vi "Test Asic Digital Offset.vi"(8 "Error IN":errorcluster, 11 "Config Test IN":T4={"Config HW"={"VISA Rigol DP832"="Rigol_DP832", "Config Rigol DP832"=[{"Channel"=0, "V Limit"=5.5, "I Limit"=0.5, "V Out"=5.0}, {"Channel"=1, "V Limit"=5.5, "I Limit"=0.8, "V Out"=5.0}, {"Channel"=2, "V Limit"=5.5, "I Limit"=0.2, "V Out"=0.0}], "CTA Test#"="CTA013 A", "FT_Handle"=0, "Espera acceso FT"=10, "VISA Tek MDO3104"="Rigol_DP832", "VISA Key 81160A"="Rigol_DP832"}, "Config Test"=[{"Vasic"=2.8, "Global Reset"=FALSE, "Test Register?"=FALSE, "Test ADC?"=FALSE, "Test ADC"={"Repeats ADC"=100, "Max Desviation"=0.1}, "Limits ADC"={"Low"=[1.9, 1.3, 0.65, 0.0, 1.6, 1.4, 1.4, 0.9, 2.1, 0.85, 1.9], "High"=[2.1, 1.5, 0.85, 0.1, 1.4, 1.2, 1.2, 0.7, 1.9, 0.65, 1.7]}, "Test Max PN Min NP?"=FALSE, "Limits Max PN Min NP"={"Max P Upper"=2.177000045776367, "Min P Upper"=1.474, "Max N Upper"=1.475, "Min N Upper"=0.818, "Max P Lower"=1.888, "Min P Lower "=1.321, "Max N Lower"=1.322, "Min N Lower"=0.73}, "Test Rate Scan?"=FALSE, "Vin Rate Scan"=[], "Limits Rate Scan"={"High"=[0.15, 0.242, 0.331, 0.425, 0.512, 0.6, 0.688, 0.774, 0.847, 0.91], "Low"=[0.021, 0.11, 0.189, 0.27, 0.347, 0.421, 0.487, 0.551, 0.601, 0.635]}, "Test Rate Scan Adders?"=FALSE, "Vin Rate Adders"=[], "Limits Rate Scan adders"={"High"=[], "Low"=[]}, "Test offset analog?"=FALSE, "Lim Offset Analog"={"Max Analog"=0.05, "Min Analog"=-0.05}, "Test offset digital?"=FALSE, "Lim offset Dig"={"Max Dig"=0.05}, "Vasic real f.a."=2.8, "IBIAS"=FALSE, "VALUE IBIAS"=63}, {"Vasic"=2.8, "Global Reset"=FALSE, "Test Register?"=FALSE, "Test ADC?"=FALSE, "Test ADC"={"Repeats ADC"=100, "Max Desviation"=0.1}, "Limits ADC"={"Low"=[1.9, 1.3, 0.65, 0.0, 1.6, 1.4, 1.4, 0.9, 2.1, 0.85, 1.9], "High"=[2.1, 1.5, 0.85, 0.1, 1.4, 1.2, 1.2, 0.7, 1.9, 0.65, 1.7]}, "Test Max PN Min NP?"=FALSE, "Limits Max PN Min NP"={"Max P Upper"=2.177000045776367, "Min P Upper"=1.474, "Max N Upper"=1.475, "Min N Upper"=0.818, "Max P Lower"=1.888, "Min P Lower "=1.321, "Max N Lower"=1.322, "Min N Lower"=0.73}, "Test Rate Scan?"=FALSE, "Vin Rate Scan"=[], "Limits Rate Scan"={"High"=[0.15, 0.242, 0.331, 0.425, 0.512, 0.6, 0.688, 0.774, 0.847, 0.91], "Low"=[0.021, 0.11, 0.189, 0.27, 0.347, 0.421, 0.487, 0.551, 0.601, 0.635]}, "Test Rate Scan Adders?"=FALSE, "Vin Rate Adders"=[], "Limits Rate Scan adders"={"High"=[], "Low"=[]}, "Test offset analog?"=FALSE, "Lim Offset Analog"={"Max Analog"=0.05, "Min Analog"=-0.05}, "Test offset digital?"=FALSE, "Lim offset Dig"={"Max Dig"=0.05}, "Vasic real f.a."=2.8, "IBIAS"=FALSE, "VALUE IBIAS"=63}, {"Vasic"=2.8, "Global Reset"=FALSE, "Test Register?"=FALSE, "Test ADC?"=FALSE, "Test ADC"={"Repeats ADC"=100, "Max Desviation"=0.1}, "Limits ADC"={"Low"=[1.9, 1.3, 0.65, 0.0, 1.6, 1.4, 1.4, 0.9, 2.1, 0.85, 1.9], "High"=[2.1, 1.5, 0.85, 0.1, 1.4, 1.2, 1.2, 0.7, 1.9, 0.65, 1.7]}, "Test Max PN Min NP?"=FALSE, "Limits Max PN Min NP"={"Max P Upper"=2.177000045776367, "Min P Upper"=1.474, "Max N Upper"=1.475, "Min N Upper"=0.818, "Max P Lower"=1.888, "Min P Lower "=1.321, "Max N Lower"=1.322, "Min N Lower"=0.73}, "Test Rate Scan?"=FALSE, "Vin Rate Scan"=[], "Limits Rate Scan"={"High"=[0.15, 0.242, 0.331, 0.425, 0.512, 0.6, 0.688, 0.774, 0.847, 0.91], "Low"=[0.021, 0.11, 0.189, 0.27, 0.347, 0.421, 0.487, 0.551, 0.601, 0.635]}, "Test Rate Scan Adders?"=FALSE, "Vin Rate Adders"=[], "Limits Rate Scan adders"={"High"=[], "Low"=[]}, "Test offset analog?"=FALSE, "Lim Offset Analog"={"Max Analog"=0.05, "Min Analog"=-0.05}, "Test offset digital?"=FALSE, "Lim offset Dig"={"Max Dig"=0.05}, "Vasic real f.a."=2.8, "IBIAS"=FALSE, "VALUE IBIAS"=63}, {"Vasic"=2.8, "Global Reset"=FALSE, "Test Register?"=FALSE, "Test ADC?"=FALSE, "Test ADC"={"Repeats ADC"=100, "Max Desviation"=0.1}, "Limits ADC"={"Low"=[1.9, 1.3, 0.65, 0.0, 1.6, 1.4, 1.4, 0.9, 2.1, 0.85, 1.9], "High"=[2.1, 1.5, 0.85, 0.1, 1.4, 1.2, 1.2, 0.7, 1.9, 0.65, 1.7]}, "Test Max PN Min NP?"=FALSE, "Limits Max PN Min NP"={"Max P Upper"=2.177000045776367, "Min P Upper"=1.474, "Max N Upper"=1.475, "Min N Upper"=0.818, "Max P Lower"=1.888, "Min P Lower "=1.321, "Max N Lower"=1.322, "Min N Lower"=0.73}, "Test Rate Scan?"=FALSE, "Vin Rate Scan"=[], "Limits Rate Scan"={"High"=[0.15, 0.242, 0.331, 0.425, 0.512, 0.6, 0.688, 0.774, 0.847, 0.91], "Low"=[0.021, 0.11, 0.189, 0.27, 0.347, 0.421, 0.487, 0.551, 0.601, 0.635]}, "Test Rate Scan Adders?"=FALSE, "Vin Rate Adders"=[], "Limits Rate Scan adders"={"High"=[], "Low"=[]}, "Test offset analog?"=FALSE, "Lim Offset Analog"={"Max Analog"=0.05, "Min Analog"=-0.05}, "Test offset digital?"=FALSE, "Lim offset Dig"={"Max Dig"=0.05}, "Vasic real f.a."=2.8, "IBIAS"=FALSE, "VALUE IBIAS"=63}], "Result"=[], "Execucion Test"={"Vasic Actual"=0}, "Config VGA"={"Theoretical Voltage"=[], "Real Voltage"=[102.85, 207.14, 299.57, 404.85, 495.71, 606.85, 697.71, 801.14, 897.14, 998.85], "Pulse Width"=57344, "Frecuency Pulse"=1000000.0, "VGA Gain"=[9, 16, 24, 34, 43, 52, 61, 72, 81, 93]}, "Test Info"={"Asic"="", "Operator"="", "Place"="", "Time start"=timestamp(0 s since 1904-01-01), "Time stop"=timestamp(0 s since 1904-01-01)}, "Info machine"={"SO"="", "SO Name"="", "SO Ver"="", "SO Build"="", "CPU"="", "APP"="", "APP YEAR"="", "APP ver"="", "APP User"="", "APP Serail"="", "MAC"=[], "PC NAME"=[], "PC IP"=[], "BIOS MANU"="", "BIOS NAME"="", "BIOS SERIAL"="", "BOARD MANU"="", "BOARD NAME"="", "BOARD SERIAL"="", "Driver Version"="", "Library Version"="", "FPGA Ver"=0, "ID CTA board"=0, "LAST BOOT"="", "LABVIEW Ver"=0}, "Partial Report"="", "CONFIG GEN"=[]} {"CONFIG GEN"."Vasic Theorical" min=1.0 max=1000000.0 step=1.0 format="%#_6pV"; "CONFIG GEN"."Frequency" min=0.001 max=333000000.0 step=1000.0 format="%#_6pHz"; "CONFIG GEN"."Leading Edge Time" min=1e-09 max=1.0 step=1e-10 format="%#_6ps"; "CONFIG GEN"."Trailing Edge Time" min=1e-09 max=1.0 step=1e-10 format="%#_6ps"; "CONFIG GEN"."Delay" min=0.0 max=1.0 step=1e-12 format="%#_6ps"; "CONFIG GEN"."Trigger Level Sync" items=["ECL", "TTL"]; "CONFIG GEN"."Trigger Sync Out" items=["AB"=3, "B"=2, "A"=1, "None"=0]; "CONFIG GEN"."Load" min=1.0 max=1000000.0 step=1.0 format="%#_6p"; "CONFIG GEN"."DC Offset" min=-10.0 max=10.0 step=0.1 format="%#_6pV"; "CONFIG GEN"."Amplitude" min=0.05 max=5.0 step=0.001 format="%#_6pV"; "CONFIG GEN"."Width Time" min=1.5e-09 max=1.0 step=1e-10 format="%#_6ps"; "CONFIG GEN"."Channel" items=["Channel1"=1, "Channel2"=2]; "Config VGA"."Theoretical Voltage" format="%1.4f"; "Config VGA"."VGA Gain" format="%02x"; "Config VGA"."Frecuency Pulse" format="%0_2p"; "Config VGA"."Pulse Width" format="%04x"; "Config VGA"."Real Voltage" format="%1.5f"; "Config Test"."VALUE IBIAS" max=63 step=1; "Config Test"."Vasic real f.a." min=2.8 max=3.8 step=0.01 format="%.2g"; "Config Test"."Limits Rate Scan adders"."Low" format="%1.3f"; "Config Test"."Limits Rate Scan adders"."High" format="%1.3f"; "Config Test"."Limits ADC"."High" format="%1.4f"; "Config Test"."Limits ADC"."Low" format="%1.3f"; "Config Test"."Lim offset Dig"."Max Dig" format="%.3g"; "Config Test"."Lim Offset Analog"."Min Analog" format="%.3g"; "Config Test"."Lim Offset Analog"."Max Analog" format="%.3g"; "Config Test"."Limits Rate Scan"."Low" format="%1.4f"; "Config Test"."Limits Rate Scan"."High" format="%1.3f"; "Config Test"."Limits Max PN Min NP"."Min P Upper" format="%.3g"; "Config Test"."Limits Max PN Min NP"."Min P Lower" format="%.3g"; "Config Test"."Limits Max PN Min NP"."Max N Lower" format="%.3g"; "Config Test"."Limits Max PN Min NP"."Max N Upper" format="%.3g"; "Config Test"."Limits Max PN Min NP"."Min N Lower" format="%.3g"; "Config Test"."Limits Max PN Min NP"."Min N Upper" format="%.3g"; "Config Test"."Limits Max PN Min NP"."Max P Upper" format="%.3g"; "Config Test"."Limits Max PN Min NP"."Max P Lower" format="%.3g"; "Config Test"."Vasic" min=2.8 max=3.8 step=0.01 format="%.2g"; "Config HW"."Config Rigol DP832"."Channel" items=["+30V Channel 1", "+30V Channel 2", "+5V Channel 3"]; "Config HW"."Config Rigol DP832"."V Limit" format="%.1g"; "Config HW"."Config Rigol DP832"."I Limit" format="%.1g"; "Config HW"."Config Rigol DP832"."V Out" format="%.1g"; "Result"."Test Registros"."Read W/R" format="%04x"; "Result"."Test Registros"."Pattern W/R" format="%04x"; "Result"."Test Registros"."Read Default" format="%04x"; "Result"."Test Registros"."Pattern Default" format="%04x"}) -> (0 "Error OUT":errorcluster, 2 "digital offset all ok":bool, 3 "Config Test OUT":T4={"Config HW"={"VISA Rigol DP832"="Rigol_DP832", "Config Rigol DP832"=[{"Channel"=0, "V Limit"=5.5, "I Limit"=0.5, "V Out"=5.0}, {"Channel"=1, "V Limit"=5.5, "I Limit"=0.8, "V Out"=5.0}, {"Channel"=2, "V Limit"=5.5, "I Limit"=0.2, "V Out"=0.0}], "CTA Test#"="CTA013 A", "FT_Handle"=0, "Espera acceso FT"=10, "VISA Tek MDO3104"="Rigol_DP832", "VISA Key 81160A"="Rigol_DP832"}, "Config Test"=[{"Vasic"=2.8, "Global Reset"=FALSE, "Test Register?"=FALSE, "Test ADC?"=FALSE, "Test ADC"={"Repeats ADC"=100, "Max Desviation"=0.1}, "Limits ADC"={"Low"=[1.9, 1.3, 0.65, 0.0, 1.6, 1.4, 1.4, 0.9, 2.1, 0.85, 1.9], "High"=[2.1, 1.5, 0.85, 0.1, 1.4, 1.2, 1.2, 0.7, 1.9, 0.65, 1.7]}, "Test Max PN Min NP?"=FALSE, "Limits Max PN Min NP"={"Max P Upper"=2.177000045776367, "Min P Upper"=1.474, "Max N Upper"=1.475, "Min N Upper"=0.818, "Max P Lower"=1.888, "Min P Lower "=1.321, "Max N Lower"=1.322, "Min N Lower"=0.73}, "Test Rate Scan?"=FALSE, "Vin Rate Scan"=[], "Limits Rate Scan"={"High"=[0.15, 0.242, 0.331, 0.425, 0.512, 0.6, 0.688, 0.774, 0.847, 0.91], "Low"=[0.021, 0.11, 0.189, 0.27, 0.347, 0.421, 0.487, 0.551, 0.601, 0.635]}, "Test Rate Scan Adders?"=FALSE, "Vin Rate Adders"=[], "Limits Rate Scan adders"={"High"=[], "Low"=[]}, "Test offset analog?"=FALSE, "Lim Offset Analog"={"Max Analog"=0.05, "Min Analog"=-0.05}, "Test offset digital?"=FALSE, "Lim offset Dig"={"Max Dig"=0.05}, "Vasic real f.a."=2.8, "IBIAS"=FALSE, "VALUE IBIAS"=63}, {"Vasic"=2.8, "Global Reset"=FALSE, "Test Register?"=FALSE, "Test ADC?"=FALSE, "Test ADC"={"Repeats ADC"=100, "Max Desviation"=0.1}, "Limits ADC"={"Low"=[1.9, 1.3, 0.65, 0.0, 1.6, 1.4, 1.4, 0.9, 2.1, 0.85, 1.9], "High"=[2.1, 1.5, 0.85, 0.1, 1.4, 1.2, 1.2, 0.7, 1.9, 0.65, 1.7]}, "Test Max PN Min NP?"=FALSE, "Limits Max PN Min NP"={"Max P Upper"=2.177000045776367, "Min P Upper"=1.474, "Max N Upper"=1.475, "Min N Upper"=0.818, "Max P Lower"=1.888, "Min P Lower "=1.321, "Max N Lower"=1.322, "Min N Lower"=0.73}, "Test Rate Scan?"=FALSE, "Vin Rate Scan"=[], "Limits Rate Scan"={"High"=[0.15, 0.242, 0.331, 0.425, 0.512, 0.6, 0.688, 0.774, 0.847, 0.91], "Low"=[0.021, 0.11, 0.189, 0.27, 0.347, 0.421, 0.487, 0.551, 0.601, 0.635]}, "Test Rate Scan Adders?"=FALSE, "Vin Rate Adders"=[], "Limits Rate Scan adders"={"High"=[], "Low"=[]}, "Test offset analog?"=FALSE, "Lim Offset Analog"={"Max Analog"=0.05, "Min Analog"=-0.05}, "Test offset digital?"=FALSE, "Lim offset Dig"={"Max Dig"=0.05}, "Vasic real f.a."=2.8, "IBIAS"=FALSE, "VALUE IBIAS"=63}, {"Vasic"=2.8, "Global Reset"=FALSE, "Test Register?"=FALSE, "Test ADC?"=FALSE, "Test ADC"={"Repeats ADC"=100, "Max Desviation"=0.1}, "Limits ADC"={"Low"=[1.9, 1.3, 0.65, 0.0, 1.6, 1.4, 1.4, 0.9, 2.1, 0.85, 1.9], "High"=[2.1, 1.5, 0.85, 0.1, 1.4, 1.2, 1.2, 0.7, 1.9, 0.65, 1.7]}, "Test Max PN Min NP?"=FALSE, "Limits Max PN Min NP"={"Max P Upper"=2.177000045776367, "Min P Upper"=1.474, "Max N Upper"=1.475, "Min N Upper"=0.818, "Max P Lower"=1.888, "Min P Lower "=1.321, "Max N Lower"=1.322, "Min N Lower"=0.73}, "Test Rate Scan?"=FALSE, "Vin Rate Scan"=[], "Limits Rate Scan"={"High"=[0.15, 0.242, 0.331, 0.425, 0.512, 0.6, 0.688, 0.774, 0.847, 0.91], "Low"=[0.021, 0.11, 0.189, 0.27, 0.347, 0.421, 0.487, 0.551, 0.601, 0.635]}, "Test Rate Scan Adders?"=FALSE, "Vin Rate Adders"=[], "Limits Rate Scan adders"={"High"=[], "Low"=[]}, "Test offset analog?"=FALSE, "Lim Offset Analog"={"Max Analog"=0.05, "Min Analog"=-0.05}, "Test offset digital?"=FALSE, "Lim offset Dig"={"Max Dig"=0.05}, "Vasic real f.a."=2.8, "IBIAS"=FALSE, "VALUE IBIAS"=63}, {"Vasic"=2.8, "Global Reset"=FALSE, "Test Register?"=FALSE, "Test ADC?"=FALSE, "Test ADC"={"Repeats ADC"=100, "Max Desviation"=0.1}, "Limits ADC"={"Low"=[1.9, 1.3, 0.65, 0.0, 1.6, 1.4, 1.4, 0.9, 2.1, 0.85, 1.9], "High"=[2.1, 1.5, 0.85, 0.1, 1.4, 1.2, 1.2, 0.7, 1.9, 0.65, 1.7]}, "Test Max PN Min NP?"=FALSE, "Limits Max PN Min NP"={"Max P Upper"=2.177000045776367, "Min P Upper"=1.474, "Max N Upper"=1.475, "Min N Upper"=0.818, "Max P Lower"=1.888, "Min P Lower "=1.321, "Max N Lower"=1.322, "Min N Lower"=0.73}, "Test Rate Scan?"=FALSE, "Vin Rate Scan"=[], "Limits Rate Scan"={"High"=[0.15, 0.242, 0.331, 0.425, 0.512, 0.6, 0.688, 0.774, 0.847, 0.91], "Low"=[0.021, 0.11, 0.189, 0.27, 0.347, 0.421, 0.487, 0.551, 0.601, 0.635]}, "Test Rate Scan Adders?"=FALSE, "Vin Rate Adders"=[], "Limits Rate Scan adders"={"High"=[], "Low"=[]}, "Test offset analog?"=FALSE, "Lim Offset Analog"={"Max Analog"=0.05, "Min Analog"=-0.05}, "Test offset digital?"=FALSE, "Lim offset Dig"={"Max Dig"=0.05}, "Vasic real f.a."=2.8, "IBIAS"=FALSE, "VALUE IBIAS"=63}], "Result"=[], "Execucion Test"={"Vasic Actual"=0}, "Config VGA"={"Theoretical Voltage"=[], "Real Voltage"=[102.85, 207.14, 299.57, 404.85, 495.71, 606.85, 697.71, 801.14, 897.14, 998.85], "Pulse Width"=57344, "Frecuency Pulse"=1000000.0, "VGA Gain"=[9, 16, 24, 34, 43, 52, 61, 72, 81, 93]}, "Test Info"={"Asic"="", "Operator"="", "Place"="", "Time start"=timestamp(0 s since 1904-01-01), "Time stop"=timestamp(0 s since 1904-01-01)}, "Info machine"={"SO"="", "SO Name"="", "SO Ver"="", "SO Build"="", "CPU"="", "APP"="", "APP YEAR"="", "APP ver"="", "APP User"="", "APP Serail"="", "MAC"=[], "PC NAME"=[], "PC IP"=[], "BIOS MANU"="", "BIOS NAME"="", "BIOS SERIAL"="", "BOARD MANU"="", "BOARD NAME"="", "BOARD SERIAL"="", "Driver Version"="", "Library Version"="", "FPGA Ver"=0, "ID CTA board"=0, "LAST BOOT"="", "LABVIEW Ver"=0}, "Partial Report"="", "CONFIG GEN"=[]} {"CONFIG GEN"."Vasic Theorical" min=1.0 max=1000000.0 step=1.0 format="%#_6pV"; "CONFIG GEN"."Frequency" min=0.001 max=333000000.0 step=1000.0 format="%#_6pHz"; "CONFIG GEN"."Leading Edge Time" min=1e-09 max=1.0 step=1e-10 format="%#_6ps"; "CONFIG GEN"."Trailing Edge Time" min=1e-09 max=1.0 step=1e-10 format="%#_6ps"; "CONFIG GEN"."Delay" min=0.0 max=1.0 step=1e-12 format="%#_6ps"; "CONFIG GEN"."Trigger Level Sync" items=["ECL", "TTL"]; "CONFIG GEN"."Trigger Sync Out" items=["AB"=3, "B"=2, "A"=1, "None"=0]; "CONFIG GEN"."Load" min=1.0 max=1000000.0 step=1.0 format="%#_6p"; "CONFIG GEN"."DC Offset" min=-10.0 max=10.0 step=0.1 format="%#_6pV"; "CONFIG GEN"."Amplitude" min=0.05 max=5.0 step=0.001 format="%#_6pV"; "CONFIG GEN"."Width Time" min=1.5e-09 max=1.0 step=1e-10 format="%#_6ps"; "CONFIG GEN"."Channel" items=["Channel1"=1, "Channel2"=2]; "Config VGA"."Theoretical Voltage" format="%1.4f"; "Config VGA"."VGA Gain" format="%02x"; "Config VGA"."Frecuency Pulse" format="%0_2p"; "Config VGA"."Pulse Width" format="%04x"; "Config VGA"."Real Voltage" format="%1.5f"; "Config Test"."VALUE IBIAS" max=63 step=1; "Config Test"."Vasic real f.a." min=2.8 max=3.8 step=0.01 format="%.2g"; "Config Test"."Limits Rate Scan adders"."Low" format="%1.3f"; "Config Test"."Limits Rate Scan adders"."High" format="%1.3f"; "Config Test"."Limits ADC"."High" format="%1.4f"; "Config Test"."Limits ADC"."Low" format="%1.3f"; "Config Test"."Lim offset Dig"."Max Dig" format="%.3g"; "Config Test"."Lim Offset Analog"."Min Analog" format="%.3g"; "Config Test"."Lim Offset Analog"."Max Analog" format="%.3g"; "Config Test"."Limits Rate Scan"."Low" format="%1.4f"; "Config Test"."Limits Rate Scan"."High" format="%1.3f"; "Config Test"."Limits Max PN Min NP"."Min P Upper" format="%.3g"; "Config Test"."Limits Max PN Min NP"."Min P Lower" format="%.3g"; "Config Test"."Limits Max PN Min NP"."Max N Lower" format="%.3g"; "Config Test"."Limits Max PN Min NP"."Max N Upper" format="%.3g"; "Config Test"."Limits Max PN Min NP"."Min N Lower" format="%.3g"; "Config Test"."Limits Max PN Min NP"."Min N Upper" format="%.3g"; "Config Test"."Limits Max PN Min NP"."Max P Upper" format="%.3g"; "Config Test"."Limits Max PN Min NP"."Max P Lower" format="%.3g"; "Config Test"."Vasic" min=2.8 max=3.8 step=0.01 format="%.2g"; "Config HW"."Config Rigol DP832"."Channel" items=["+30V Channel 1", "+30V Channel 2", "+5V Channel 3"]; "Config HW"."Config Rigol DP832"."V Limit" format="%.1g"; "Config HW"."Config Rigol DP832"."I Limit" format="%.1g"; "Config HW"."Config Rigol DP832"."V Out" format="%.1g"; "Result"."Test Registros"."Read W/R" format="%04x"; "Result"."Test Registros"."Pattern W/R" format="%04x"; "Result"."Test Registros"."Read Default" format="%04x"; "Result"."Test Registros"."Pattern Default" format="%04x"})   [LabVIEW 2019]
uses:
  Test.ctl
  TEST.TEST CONFIG HW.ctl
  Rigol DP832/DP832_Control Channels.ctl
  TEST.TEST CONFIG TEST MATRIZ.ctl
  TEST.TEST CONFIG TEST.ctl
  TEST.TEST RESULT.ctl
  test_result fvasic.ctl
  TEST.TEST EXECUTION TEST.ctl
  TEST.TEST CONFIG VGA.ctl
  TEST.TEST TEST INFO.ctl
  TEST.TEST INFO PC.ctl
  GenPulse_configurar.ctl
  ASIC.digital offset start-stop.ctl
  Global.Salir Ya.vi
panel:
  in  "Tab Control":enum32{"Page 1", "Page 2"}(tab)
  out "%":u8 format="%02d%%"
  out "B":u8(slide) scale=0.0..100.0
  out "Indicador":string
  out "Result":T1 {"Test Registros"."Read W/R" format="%04x"; "Test Registros"."Pattern W/R" format="%04x"; "Test Registros"."Read Default" format="%04x"; "Test Registros"."Pattern Default" format="%04x"}
  out "VALORES START-STOP":T2
  out "Todos los valores":T3
  out "REF":cluster{"Sumador":u8, "Canal":u8}
  # "Test ASIC. Digital Offset"
  # "Modo 2\nModo 3\nModo 4\nModo 2\nModo 3\nModo 4"
  # "Modo 2\nModo 3\nModo 4\nModo 2\nModo 3\nModo 4"
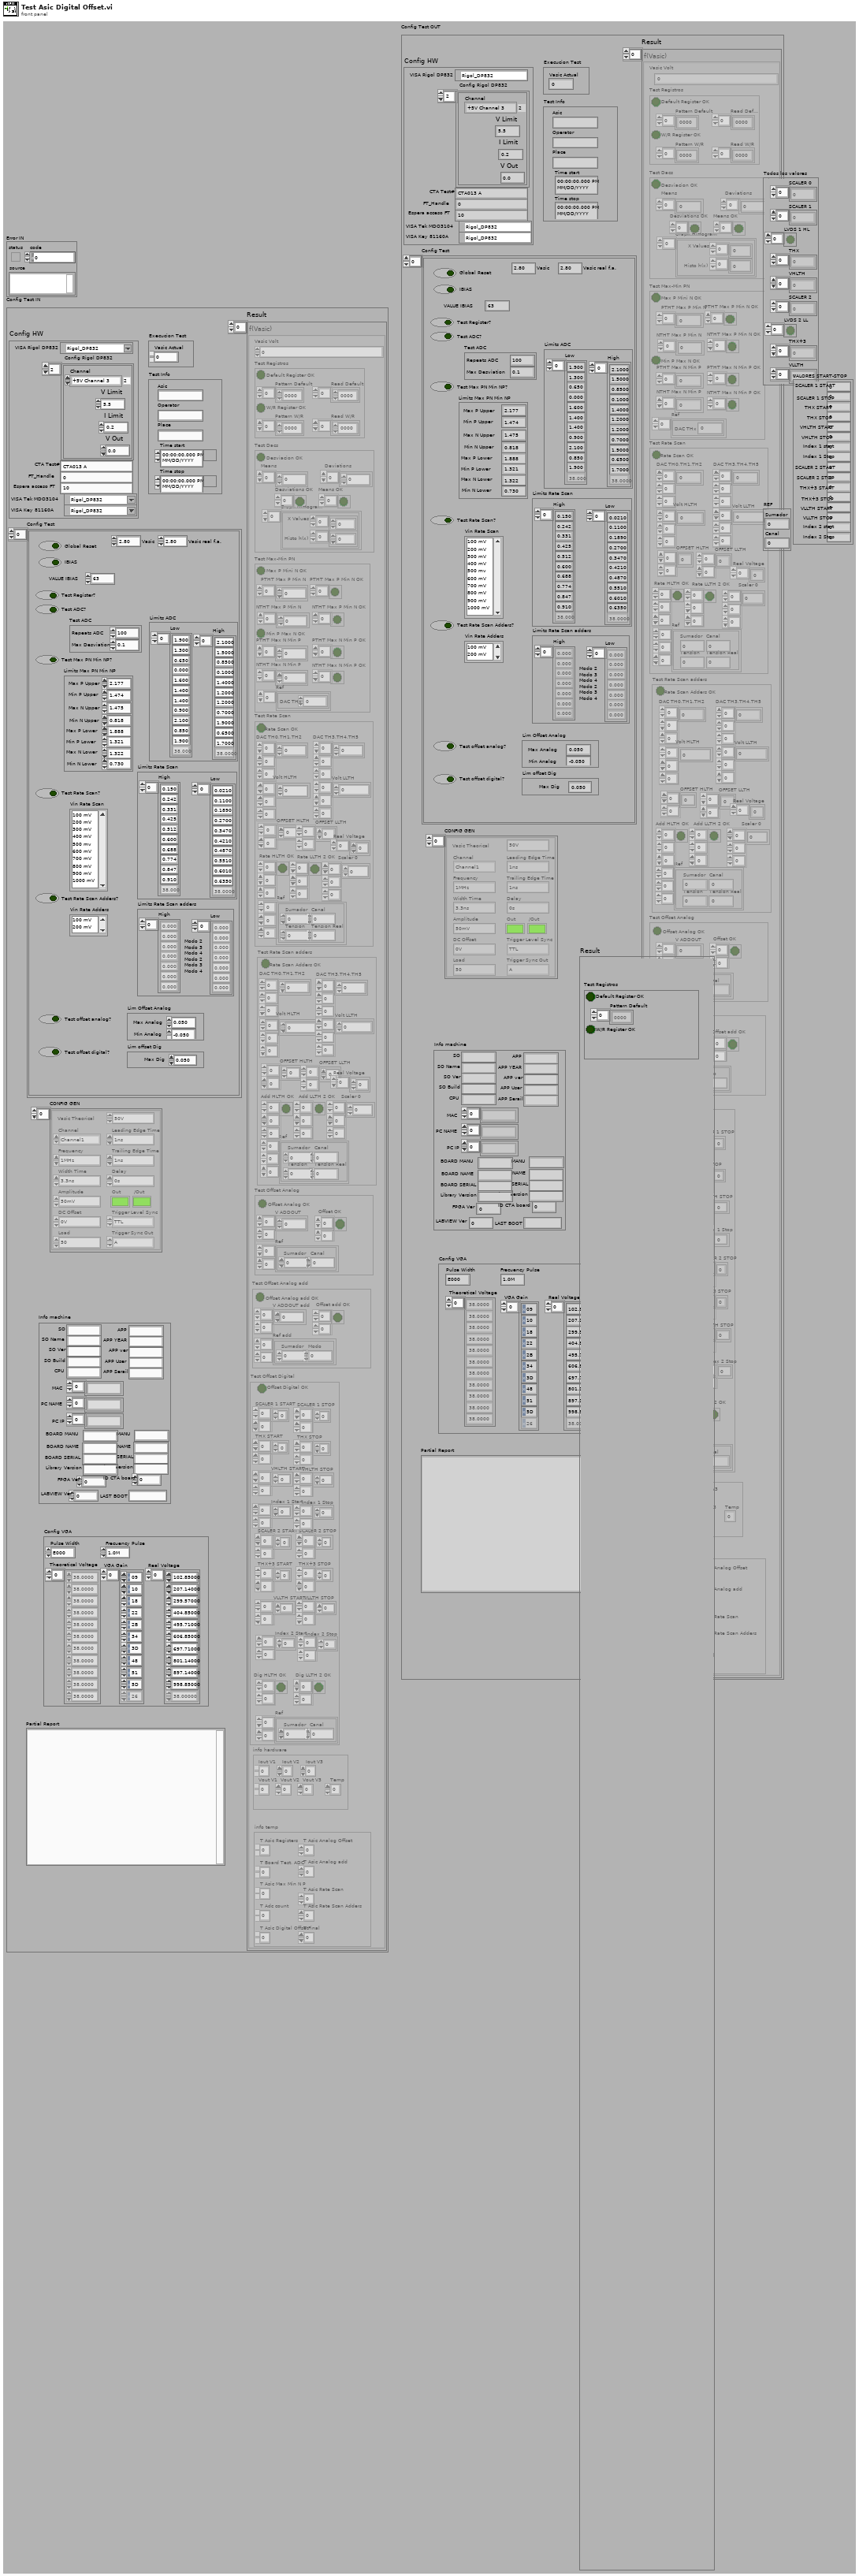
[diagram p1: front panel]
types:
  T1 = typedef "test_result fvasic.ctl" = cluster{"Vasic Volt":i32, "Test Registros":cluster{"Default Register OK":bool, "Pattern Default":u16[], "Read Default":u16[], "W/R Register OK":bool, "Pattern W/R":u16[], "Read W/R":u16[]}, "Test Dacs":cluster{"Desviacion OK":bool, "Means":dbl[], "Deviations":dbl[], "Desviations OK":bool[], "Means OK":bool[], "Graph Histogram":cluster{"X Values":dbl[], "Histo h(x)":i32[]}[]}, "Test Max-Min PN":cluster{"Max P Mini N OK":bool, "PTHT Max P Min N":dbl[], "PTHT Max P Min N OK":bool[], "NTHT Max P Min N":dbl[], "NTHT Max P Min N OK":bool[], "Min P Max N OK":bool, "PTHT Max N Min P":dbl[], "PTHT Max N Min P OK":bool[], "NTHT Max N Min P":dbl[], "NTHT Max N Min P OK":bool[], "Ref":cluster{"DAC THx":u8}[]}, "Test Rate Scan":cluster{"Rate Scan OK":bool, "DAC TH0,TH1,TH2":u16[][][], "Volt HLTH":dbl[][][], "Rate HLTH OK":bool[][][], "DAC TH3,TH4,TH5":u16[][][], "Volt LLTH":dbl[][][], "Rate LLTH 2 OK":bool[][][], "Scaler 0":u16[][][], "Ref":cluster{"Sumador":u8, "Canal":u8, "Tension":u8, "Tension Real":dbl}[][][], "OFFSET HLTH":dbl[][], "OFFSET LLTH":dbl[][], "Real Voltage":dbl[]}, "Test Rate Scan adders":cluster{"Rate Scan Adders OK":bool, "DAC TH0,TH1,TH2":u16[][][], "Volt HLTH":dbl[][][], "Add HLTH OK":bool[][][], "DAC TH3,TH4,TH5":u16[][][], "Volt LLTH":dbl[][][], "Add LLTH 2 OK":bool[][][], "Scaler 0":u16[][][], "Ref":cluster{"Sumador":u8, "Canal":u8, "Tension":u8, "Tension Real":dbl}[][][], "OFFSET HLTH":dbl[][], "OFFSET LLTH":dbl[][], "Real Voltage":dbl[]}, "Test Offset Analog":cluster{"Offset Analog OK":bool, "V ADDOUT":dbl[][], "Offset OK":bool[][], "Ref":cluster{"Sumador":u8, "Canal":u8}[][]}, "Test Offset Digital":cluster{"Offset Digital OK":bool, "SCALER 1 START":u16[][], "SCALER 1 STOP":u16[][], "THX START":u16[][], "THX STOP":u16[][], "VHLTH START":dbl[][], "VHLTH STOP":dbl[][], "Index 1 Start":i32[][], "index 1 Stop":i32[][], "SCALER 2 START":u16[][], "SCALER 2 STOP":u16[][], "THX+3 START":u16[][], "THX+3 STOP":u16[][], "VLLTH START":dbl[][], "VLLTH STOP":dbl[][], "Index 2 Start":i32[][], "index 2 Stop":i32[][], "Dig HLTH OK":bool[][], "Dig LLTH 2 OK":bool[][], "Ref":cluster{"Sumador":u8, "Canal":u8}[][]}, "info hardware":cluster{"Iout V1":dbl, "Iout V2":dbl, "Iout V3":dbl, "Vout V1":dbl, "Vout V2":dbl, "Vout V3":dbl, "Temp":dbl}, "Test Offset Analog add":cluster{"Offset Analog add OK":bool, "V ADDOUT add":dbl[][], "Offset add OK":bool[][], "Ref add":cluster{"Sumador":u8, "Modo":u8}[][]}, "info temp":cluster{"T Asic Registers":dbl, "T Board Test. ADC":dbl, "T Asic Max Min N P":dbl, "T Adc count":dbl, "T Asic Digital Offset":dbl, "T Asic Analog Offset":dbl, "T Asic Analog add":dbl, "T Asic Rate Scan":dbl, "T Asic Rate Scan Adders":dbl, "T Final":dbl}}
  T2 = typedef "ASIC.digital offset start-stop.ctl" = cluster{"SCALER 1 START":u16, "SCALER 1 STOP":u16, "THX START":u16, "THX STOP":u16, "VHLTH START":dbl, "VHLTH STOP":dbl, "Index 1 start":i32, "Index 1 Stop":i32, "SCALER 2 START":u16, "SCALER 2 STOP":u16, "THX+3 START":u16, "THX+3 STOP":u16, "VLLTH START":dbl, "VLLTH STOP":dbl, "Index 2 start":i32, "Index 2 Stop":i32}
  T3 = cluster{"SCALER 0":u16[], "SCALER 1":u16[], "LVDS 1 HL":bool[], "THX":u16[], "VHLTH":dbl[], "SCALER 2":u16[], "LVDS 2 LL":bool[], "THX+3":u16[], "VLLTH":dbl[]}
  T4 = typedef "Test.ctl" = cluster{"Config HW":T5, "Config Test":T7, "Result":T9, "Execucion Test":T10, "Config VGA":T11, "Test Info":T12, "Info machine":T13, "Partial Report":string, "CONFIG GEN":T14[]}
  T5 = typedef "TEST.TEST CONFIG HW.ctl" = cluster{"VISA Rigol DP832":refnum<visa-resource-name>, "Config Rigol DP832":cluster{"Channel":T6, "V Limit":dbl, "I Limit":dbl, "V Out":dbl}[], "CTA Test#":string, "FT_Handle":u32, "Espera acceso FT":u32, "VISA Tek MDO3104":refnum<visa-resource-name>, "VISA Key 81160A":refnum<visa-resource-name>}
  T6 = typedef "DP832_Control Channels.ctl" = i32
  T7 = typedef "TEST.TEST CONFIG TEST MATRIZ.ctl" = T8[]
  T8 = typedef "TEST.TEST CONFIG TEST.ctl" = cluster{"Vasic":dbl, "Global Reset":bool, "Test Register?":bool, "Test ADC?":bool, "Test ADC":cluster{"Repeats ADC":i32, "Max Desviation":dbl}, "Limits ADC":cluster{"Low":dbl[], "High":dbl[]}, "Test Max PN Min NP?":bool, "Limits Max PN Min NP":cluster{"Max P Upper":dbl, "Min P Upper":dbl, "Max N Upper":dbl, "Min N Upper":dbl, "Max P Lower":dbl, "Min P Lower ":dbl, "Max N Lower":dbl, "Min N Lower":dbl}, "Test Rate Scan?":bool, "Vin Rate Scan":i32[], "Limits Rate Scan":cluster{"High":dbl[], "Low":dbl[]}, "Test Rate Scan Adders?":bool, "Vin Rate Adders":i32[], "Limits Rate Scan adders":cluster{"High":dbl[], "Low":dbl[]}, "Test offset analog?":bool, "Lim Offset Analog":cluster{"Max Analog":dbl, "Min Analog":dbl}, "Test offset digital?":bool, "Lim offset Dig":cluster{"Max Dig":dbl}, "Vasic real f.a.":dbl, "IBIAS":bool, "VALUE IBIAS":u8}
  T9 = typedef "TEST.TEST RESULT.ctl" = T1[]
  T10 = typedef "TEST.TEST EXECUTION TEST.ctl" = cluster{"Vasic Actual":i32}
  T11 = typedef "TEST.TEST CONFIG VGA.ctl" = cluster{"Theoretical Voltage":dbl[], "Real Voltage":dbl[], "Pulse Width":u16, "Frecuency Pulse":dbl, "VGA Gain":u8[]}
  T12 = typedef "TEST.TEST TEST INFO.ctl" = cluster{"Asic":string, "Operator":string, "Place":string, "Time start":timestamp, "Time stop":timestamp}
  T13 = typedef "TEST.TEST INFO PC.ctl" = cluster{"SO":string, "SO Name":string, "SO Ver":string, "SO Build":string, "CPU":string, "APP":string, "APP YEAR":string, "APP ver":string, "APP User":string, "APP Serail":string, "MAC":string[], "PC NAME":string[], "PC IP":string[], "BIOS MANU":string, "BIOS NAME":string, "BIOS SERIAL":string, "BOARD MANU":string, "BOARD NAME":string, "BOARD SERIAL":string, "Driver Version":string, "Library Version":string, "FPGA Ver":u8, "ID CTA board":u64, "LAST BOOT":string, "LABVIEW Ver":u32}
  T14 = typedef "GenPulse_configurar.ctl" = cluster{"Channel":u16, "Frequency":dbl, "Width Time":dbl, "Amplitude":dbl, "DC Offset":dbl, "Load":dbl, "Leading Edge Time":dbl, "Trailing Edge Time":dbl, "Delay":dbl, "Out":bool, "/Out":bool, "Trigger Level Sync":u16, "Trigger Sync Out":u16, "Vasic Theorical":dbl}
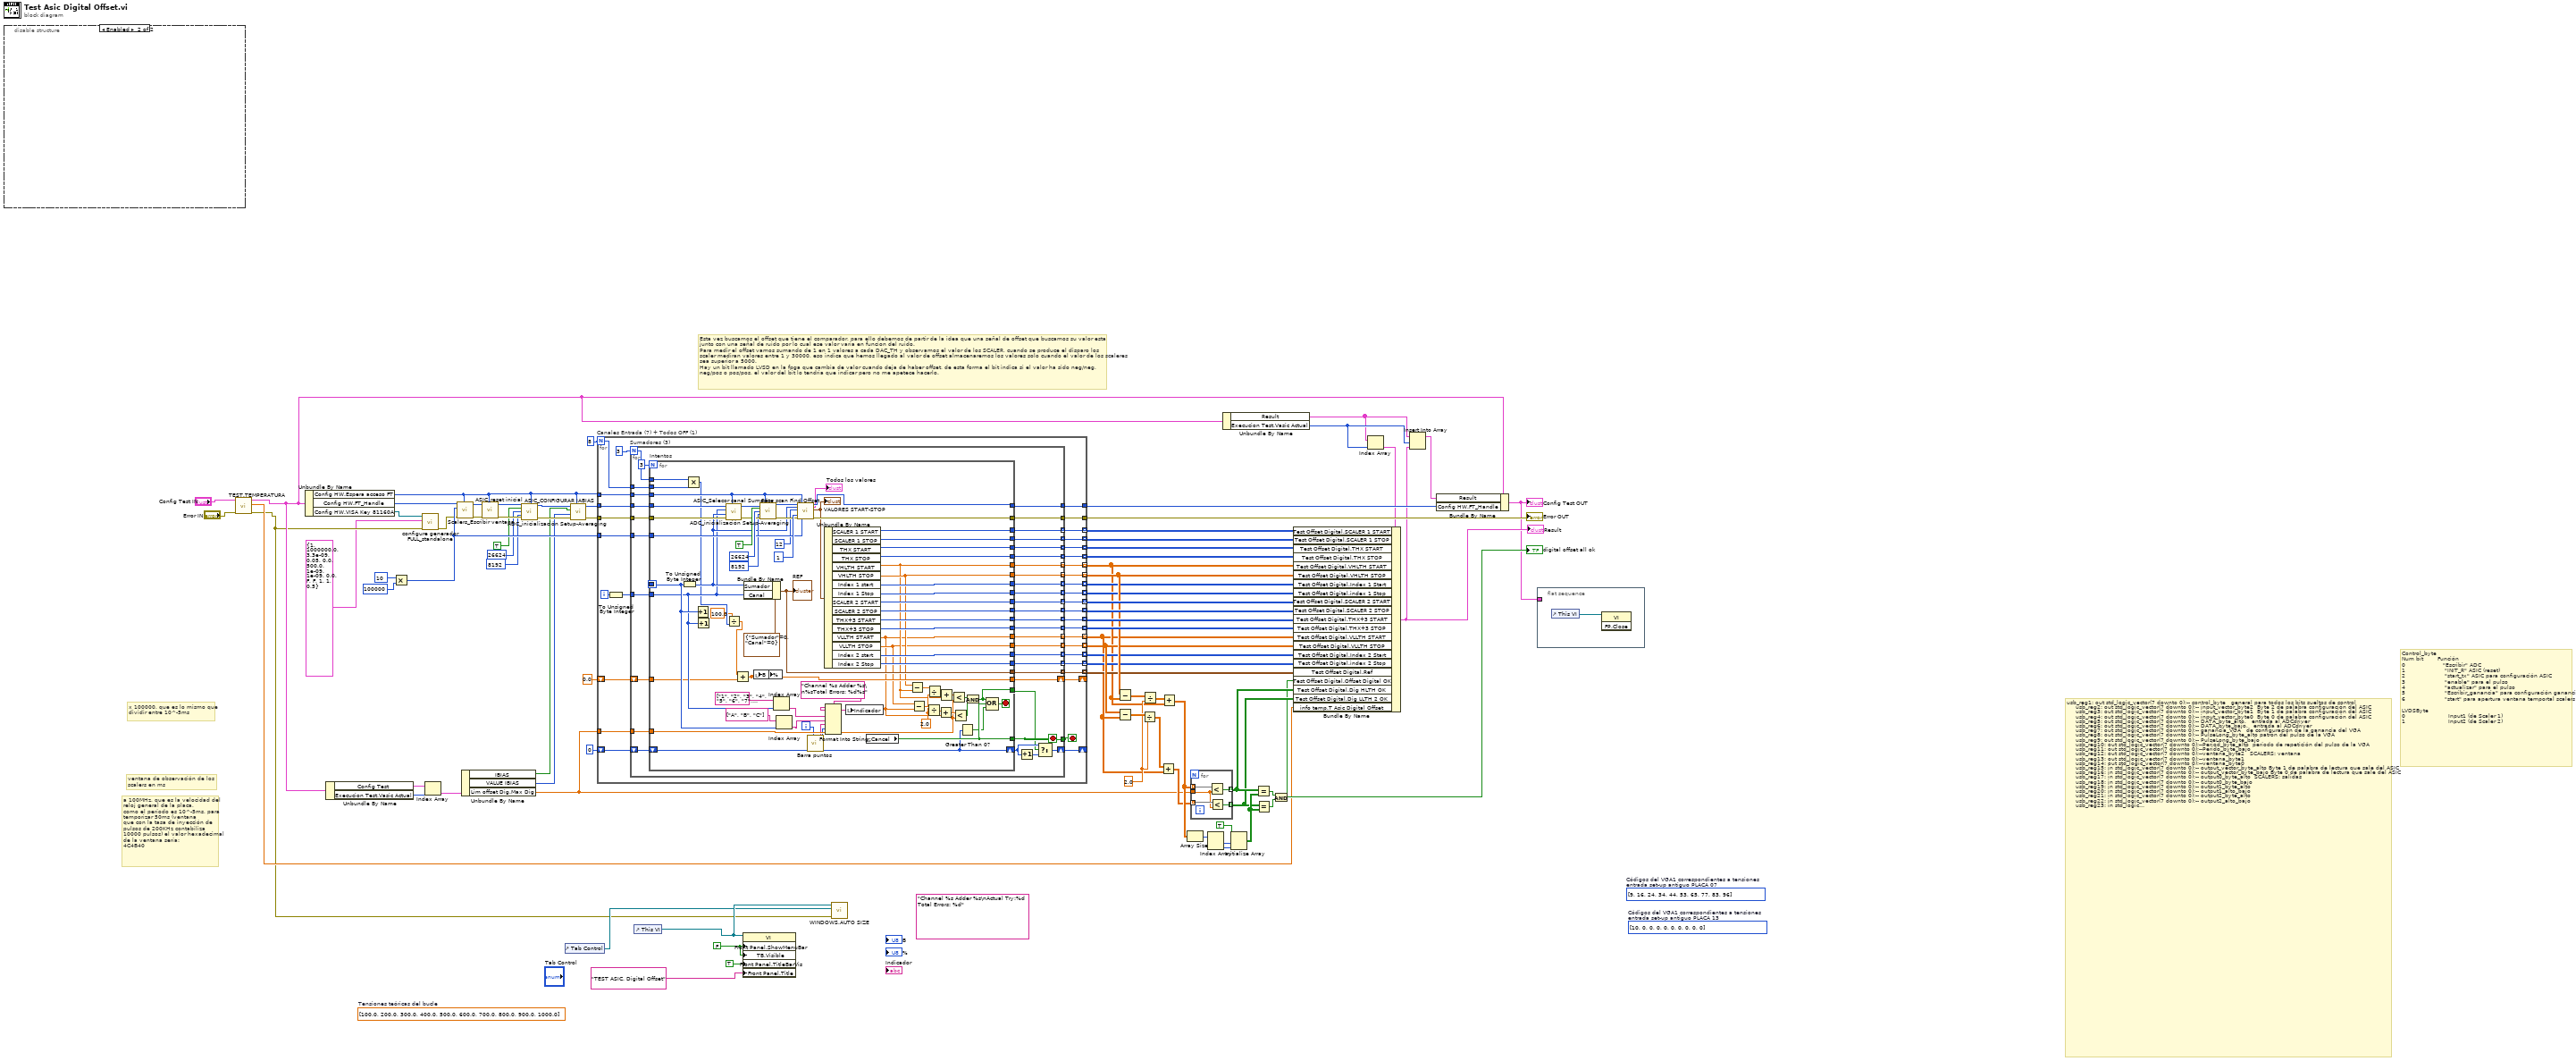
[diagram p0: block diagram]
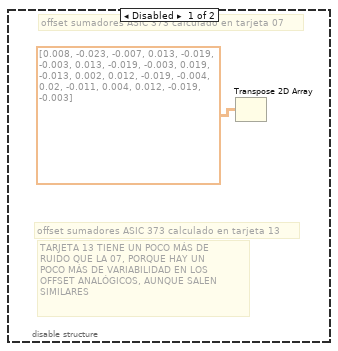
[diagram p2: hidden frame]
diagram:
  (unwired) "Channel %s Adder %s\nActual Try:%d  Total Errors: %d" ("format string")
  w26 = 2.0 ("y")
  w33 = FALSE ("Front Panel Window:Show Menu Bar")
  (unwired) dbl[] [100.0, 200.0, 300.0, 400.0, 500.0, 600.0, 700.0, 800.0, 900.0, 1000.0]  # Tensiones teóricas del bucle
  (unwired) u8[] [10, 0, 0, 0, 0, 0, 0, 0, 0, 0]  # Códigos del VGA1 correspondientes a tensiones entrada set-up antiguo PLACA 13
  (unwired) u8[] [9, 16, 24, 34, 44, 53, 65, 77, 83, 96]  # Códigos del VGA1 correspondientes a tensiones entrada set-up antiguo PLACA 07
  # "Esta vez buscamos el offset que tiene el comparador, para ello debemos de partir de la idea que una señal de offset que buscamos su valor esta\njunto con una señal de ruido por lo cual ese valor varia en funcion del ruido.\nPara medir el offset vamos sumando de 1 en 1 valores a cada DAC_TH y observamos el valor de los SCALER, cuando se produce el disparo los\nscaler mediran valores entre 1 y 30000, eso indica que hemos llegado al valor de offset almacenaremos los valores solo cuando el valor de los scaleres\nsea superior a 5000.\nHay un bit llamado LVSD en la fpga que cambia de valor cuando deja de haber offset, de esta forma el bit indica si el valor ha sido neg/neg,\nneg/pos o pos/pos, el valor del bit lo tendria que indicar pero no me apetece hacerlo."
  # "Control_byte\nNum bit        Función\n0                     \"Escribir\" ADC\n1                      \"INIT_R\" ASIC (reset)\n2                      \"start_tx\" ASIC para configuración ASIC\n3                      \"enable\" para el pulso\n4                      \"actualizar\" para el pulso\n5                      \"Escribir_ganancia\" para configuración ganancia\n6                      \"start\" para apertura ventana temportal scalers\n\nLVDSByte\n0                        Input1 (de Scaler 1)\n1                        Input2 (de Scaler 2)"
  # "usb_reg1: out std_logic_vector(7 downto 0);-- control_byte\t\t\tgeneral para todos los bits sueltos de control\n\t\t\t  usb_reg2: out std_logic_vector(7 downto 0);-- input_vector_byte2 \tByte 2 de palabra configuración del ASIC\n\t\t\t  usb_reg3: out std_logic_vector(7 downto 0);-- input_vector_byte1 \tByte 1 de palabra configuración del ASIC\n\t\t\t  usb_reg4: out std_logic_vector(7 downto 0);-- input_vector_byte0 \tByte 0 de palabra configuración del ASIC\n\t\t\t  usb_reg5: out std_logic_vector(7 downto 0);-- DATA_byte_alto, \t\tentrada al ADCdriver\n\t\t\t  usb_reg6: out std_logic_vector(7 downto 0);-- DATA_byte_bajo, \t\tentrada al ADCdriver\n\t\t\t  usb_reg7: out std_logic_vector(7 downto 0);-- ganancia_VGA\t\t\tde configuración de la ganancia del VGA\n\t\t\t  usb_reg8: out std_logic_vector(7 downto 0);-- PulseLong_byte_alto\tpatrón del pulso de la VGA\n\t\t\t  usb_reg9: out std_logic_vector(7 downto 0);-- PulseLong_byte_bajo\n\t\t\t  usb_reg10: out std_logic_vector(7 downto 0);--Period_byte_alto\t\tperíodo de repetición del pulso de la VGA\n\t\t\t  usb_reg11: out std_logic_vector(7 downto 0);--Perido_byte_bajo\n\t\t\t  usb_reg12: out std_logic_vector(7 downto 0);--ventana_byte2\t\t\tSCALERS: ventana\n\t\t\t  usb_reg13: out std_logic_vector(7 downto 0);--ventana_byte1\t\n\t\t\t  usb_reg14: out std_logic_vector(7 downto 0);--ventana_byte0\n\t\t\t  usb_reg15: in std_logic_vector(7 downto 0);-- output_vector_byte_alto\tByte 1 de palabra de lectura que sale del ASIC\n\t\t\t  usb_reg16: in std_logic_vector(7 downto 0);-- output_vector_byte_bajo\tByte 0 de palabra de lectura que sale del ASIC\n\t\t\t  usb_reg17: in std_logic_vector(7 downto 0);-- output0_byte_alto\t\tSCALERS: salidas\n\t\t\t  usb_reg18: in std_logic_vector(7 downto 0);-- output0_byte_bajo\n\t\t\t  usb_reg19: in std_logic_vector(7 downto 0);-- output1_byte_alto\n\t\t\t  usb_reg20: in std_logic_vector(7 downto 0);-- output1_alto_bajo \n\t\t\t  usb_reg21: in std_logic_vector(7 downto 0);-- output2_byte_alto \n\t\t\t  usb_reg22: in std_logic_vector(7 downto 0);-- output2_alto_bajo \n\t\t\t  usb_reg23: in std_logic_vector(7 downto 0);-- para el canal_0 del ADCdriver\n\t\t\t  usb_reg24: in std_logic_vector(7 downto 0);\n\t\t\t  usb_reg25: in std_logic_vector(7 downto 0);-- para el canal_1 del ADCdriver\n\t\t\t  usb_reg26: in std_logic_vector(7 downto 0);\n\t\t\t  usb_reg27: in std_logic_vector(7 downto 0);-- para el canal_2 del ADCdriver\n\t\t\t  usb_reg28: in std_logic_vector(7 downto 0);\n\t\t\t  usb_reg29: in std_logic_vector(7 downto 0);-- para el canal_3 del ADCdriver\n\t\t\t  usb_reg30: in std_logic_vector(7 downto 0);\n\t\t\t  usb_reg31: in std_logic_vector(7 downto 0);-- para el canal_4 del ADCdriver\n\t\t\t  usb_reg32: in std_logic_vector(7 downto 0);\n\t\t\t  usb_reg33: in std_logic_vector(7 downto 0);-- para el canal_5 del ADCdriver\n\t\t\t  usb_reg34: in std_logic_vector(7 downto 0);\n\t\t\t  usb_reg35: in std_logic_vector(7 downto 0);-- para el canal_6 del ADCdriver\n\t\t\t  usb_reg36: in std_logic_vector(7 downto 0);\n\t\t\t  usb_reg37: in std_logic_vector(7 downto 0);-- para el canal_7 del ADCdriver\n\t\t\t  usb_reg38: in std_logic_vector(7 downto 0);\n\t\t\t  usb_reg39: in std_logic_vector(7 downto 0);-- para el canal_8 del ADCdriver\n\t\t\t  usb_reg40: in std_logic_vector(7 downto 0);\n\t\t\t  usb_reg41: in std_logic_vector(7 downto 0);-- para el canal_9 del ADCdriver\n\t\t\t  usb_reg42: in std_logic_vector(7 downto 0);\n\t\t\t  usb_reg43: in std_logic_vector(7 downto 0);-- para el canal_10 del ADCdriver\n\t\t\t  usb_reg44: in std_logic_vector(7 downto 0)--;  \n\n     usb_reg55 => LVDSByte"
  # "x 100000, que es lo mismo que dividir entre 10^-5ms"
  # "ventana de observación de los scalers en ms"
  # "a 100MHz, que es la velocidad del reloj general de la placa,\ncomo el período es 10^-5ms, para temporizar 50ms (ventana \nque con la tasa de inyección de pulsos de 200KHz contabiliza \n10000 pulsos) el valor hexadecimal de la ventana sería:\n4C4B40"
  n1 = disable-structure shown="Enabled" {
    frame Disabled {
      # "TARJETA 13 TIENE UN POCO MÁS DE \nRUIDO QUE LA 07, PORQUE HAY UN\nPOCO MÁS DE VARIABILIDAD EN LOS \nOFFSET ANALÓGICOS, AUNQUE SALEN\nSIMILARES"
      # "offset sumadores ASIC 373 calculado en tarjeta 13"
      # "offset sumadores ASIC 373 calculado en tarjeta 07"
      n2 = Transpose 2D Array(2D array=dbl[][] [[0.008, -0.023, -0.007], [0.013, -0.019, -0.003], [0.013, -0.019, -0.003], [0.019, -0.013, 0.002], [0.012, -0.019, -0.004], [0.02, -0.011, 0.004], [0.012, -0.019, -0.003]]) -> ()  [unwired: 1 out]
    }
    frame Enabled {
    }
  }
  n3 = call "TEST.TEMPERATURA.vi"("error IN"="Error IN", "input cluster"="Config Test IN") -> ("error out"=w4:errorcluster, "Temperatura"=w7:dbl, "OUT cluster 2"=w6:T4)  [unwired: 7 in]
  n4 = Unbundle By Name(w6) -> ("Config HW.Espera acceso FT"=w14:u32, "Config HW.FT_Handle"=w5:u32, "Config HW.VISA Key 81160A"=w2:refnum<visa-resource-name>)
  n5 = Unbundle By Name(w6) -> ("Config Test"=w61:T7, "Execucion Test.Vasic Actual"=w62:i32)
  n6 = Multiply(x=u32 10 ("Ventana"), y=u32 100000 ("Ventana")) -> (x*y=w76:u32)
  n7 = call "configure generador FULL_standalone.vi"("error in"=w4, "Config Pulse"=T14 {"Channel"=1, "Frequency"=1000000.0, "Width Time"=3.3e-09, "Amplitude"=0.05, "DC Offset"=0.0, "Load"=500.0, "Leading Edge Time"=1e-09, "Trailing Edge Time"=1e-09, "Delay"=0.0, "Out"=FALSE, "/Out"=FALSE, "Trigger Level Sync"=1, "Trigger Sync Out"=1, "Vasic Theorical"=0.5}, "VISA Key 81160A"=w2) -> ("error out"=w3:errorcluster)  [unwired: 6 in, 2 out]
  n8 = Index Array(array=w61, index=w62) -> (element=w60:T8)
  n9 = call "Scalers_Escribir ventana.vi"("Espera acceso USB"=w14, "error in"=w3, "Ventana"=w76, "ftHandle_in"=w5) -> ("error out"=w77:errorcluster, "ftHandle_out"=w78:u32)  [unwired: 6 in]
  n10 = Unbundle By Name(w60) -> ("IBIAS"=w13:bool, "VALUE IBIAS"=w12:u8, "Lim offset Dig.Max Dig"=w19:dbl)
  n11 = call "ASIC_reset inicial.vi"("Espera acceso USB"=w14, "error in"=w77, "ftHandle_in"=w78) -> ("error out"=w74:errorcluster, "ftHandle_out"=w75:u32)  [unwired: 7 in]
  n12 = call "ADC_inicialización Setup-Averaging.vi"("ftHandle_in 2"=w75, "Espera acceso USB"=w14, "Reset (T=reset)"=TRUE, "Registro Setup (0x6800)"=u16 26624, "Registro Averaging (0x3200)"=u16 8192 ("Registro Setup (0x6800)"), "error in 2"=w74) -> ("ftHandle_out"=w66:u32, "error out"=w16:errorcluster)  [unwired: 8 in]
  n13 = control-ref of="Tab Control"() -> (w29:refnum<vi>)
  n14 = call "ASIC_CONFIGURAR IABIAS.vi"("Espera acceso USB"=w14, "error in"=w16, "IBIAS VALUE"=w12, "IBIAS"=w13, "ftHandle_in"=w66) -> ("error out"=w15:errorcluster, "ftHandle_out"=w17:u32)  [unwired: 5 in]
  n15 = for "Canales Entrada (7) + Todos OFF (1)" {
    N: 8 -> [w88]
    tunnel: w14 -> [w110]
    tunnel: w76 -> [w111]
    tunnel: [w105] -> w38 mode=indexing
    tunnel: [w104] -> w56 mode=indexing
    tunnel: [w103] -> w55 mode=indexing
    tunnel: [w102] -> w54 mode=indexing
    tunnel: [w101] -> w53 mode=indexing
    tunnel: [w100] -> w21 mode=indexing
    tunnel: [w99] -> w48 mode=indexing
    tunnel: [w98] -> w52 mode=indexing
    tunnel: [w97] -> w51 mode=indexing
    tunnel: [w96] -> w50 mode=indexing
    tunnel: [w95] -> w49 mode=indexing
    tunnel: [w94] -> w20 mode=indexing
    tunnel: [w93] -> w47 mode=indexing
    tunnel: [w92] -> w37 mode=indexing
    tunnel: [w91] -> w36 mode=indexing
    tunnel: [w90] -> w35 mode=indexing
    tunnel: [w89] -> w34 mode=indexing
    shift-right: [w86] -> _
    shift-left: 0.0 ("value") -> [w87]
    tunnel: w19 -> [w84]
    shift-right: [w82] -> _
    shift-left: 0 -> [w83]
    tunnel: w17 -> [w114]
    tunnel: [w107] -> w72
    tunnel: w15 -> [w113]
    tunnel: [w106] -> w73
    i -> [w112]
    stop <- w85 stop-if-true
    n16 = To Unsigned Byte Integer(number=w112) -> (unsigned 8bit integer=w108:u8)
    n17 = for "Sumadores (3)" {
      N: 3 -> [w127]
      tunnel: w108 -> [w125]
      tunnel: w111 -> [w151]
      tunnel: w110 -> [w148]
      tunnel: [w145] -> w105 mode=indexing
      tunnel: [w144] -> w104 mode=indexing
      tunnel: [w143] -> w103 mode=indexing
      tunnel: [w142] -> w102 mode=indexing
      tunnel: [w141] -> w101 mode=indexing
      tunnel: [w140] -> w100 mode=indexing
      tunnel: [w139] -> w99 mode=indexing
      tunnel: [w138] -> w98 mode=indexing
      tunnel: [w137] -> w97 mode=indexing
      tunnel: [w136] -> w96 mode=indexing
      tunnel: [w135] -> w95 mode=indexing
      tunnel: [w134] -> w94 mode=indexing
      tunnel: [w133] -> w93 mode=indexing
      tunnel: [w132] -> w92 mode=indexing
      tunnel: [w131] -> w91 mode=indexing
      tunnel: [w130] -> w90 mode=indexing
      tunnel: [w129] -> w89 mode=indexing
      tunnel: w88 -> [w128]
      shift-right: [w123] -> w86
      shift-left: w87 -> [w124]
      tunnel: [w122] -> w85
      tunnel: w84 -> [w121]
      shift-right: [w116] -> w82
      shift-left: w83 -> [w119]
      tunnel: w114 -> [w149]
      tunnel: [w147] -> w107
      tunnel: w113 -> [w150]
      tunnel: [w146] -> w106
      i -> [w126]
      stop <- w122 stop-if-true
      n18 = for "Intentos" {
        N: 3 -> [_]
        tunnel: w151 -> [w214]
        tunnel: w148 -> [w209]
        tunnel: [w202] -> w145
        tunnel: [w200] -> w144
        tunnel: [w199] -> w143
        tunnel: [w198] -> w142
        tunnel: [w197] -> w141
        tunnel: [w163] -> w140
        tunnel: [w165] -> w139
        tunnel: [w196] -> w138
        tunnel: [w195] -> w137
        tunnel: [w194] -> w136
        tunnel: [w193] -> w135
        tunnel: [w161] -> w134
        tunnel: [w162] -> w133
        tunnel: [w191] -> w132
        tunnel: [w190] -> w131
        tunnel: [w189] -> w130
        tunnel: [w188] -> w129
        tunnel: w128 -> [w187]
        tunnel: w127 -> [w186]
        tunnel: w126 -> [w179]
        tunnel: w125 -> [w178]
        tunnel: w124 -> [w175]
        tunnel: [w173] -> w123
        tunnel: [w158] -> w122
        tunnel: w121 -> [w166]
        shift-right: [w154] -> w117
        shift-left: w119 -> [w154]
        tunnel: [w156] -> w115
        tunnel: w149 -> [w212]
        tunnel: [w207] -> w147
        tunnel: w150 -> [w213]
        tunnel: [w206] -> w146
        i -> [w153]
        stop <- w157 stop-if-true
        w164 = 2.0 ("y")
        n19 = To Unsigned Byte Integer(number=w179) -> (unsigned 8bit integer=w203:u8)
        n20 = Multiply(x=w186, y=w187) -> (x*y=w177:i32)
        n21 = Increment(x=w179) -> ()  [unwired: 1 out]
        n22 = Increment(x=w178) -> ()  [unwired: 1 out]
        n23 = call "ASIC_Selecor canal Sumador.vi"("Espera acceso USB"=w209, "error in"=w213, "Sumador"=w203, "Canal"=w178, "ftHandle_in"=w212) -> ("error out"=w211:errorcluster, "ftHandle_out"=w210:u32)  [unwired: 4 in, 1 out]
        n24 = Divide(x=100.0 ("value"), y=w177) -> (x/y=w174:dbl)
        n25 = Add(x=w174, y=w175) -> (x+y=w173:dbl)
        n26 = Bundle By Name(cluster=cluster{"Sumador":u8, "Canal":u8} {"Sumador"=0, "Canal"=0}, "Sumador"=w203, "Canal"=w178) -> (w202:cluster{"Sumador":u8, "Canal":u8})
        "REF" <- w202
        n27 = local write "B"(w173) -> ()
        n28 = call "ADC_inicialización Setup-Averaging.vi"("ftHandle_in 2"=w210, "Espera acceso USB"=w209, "Reset (T=reset)"=TRUE, "Registro Setup (0x6800)"=u16 26624, "Registro Averaging (0x3200)"=u16 8192 ("Registro Setup (0x6800)"), "error in 2"=w211) -> ("ftHandle_out"=w216:u32, "error out"=w215:errorcluster)  [unwired: 8 in]
        n29 = local write "%"(w173) -> ()
        n30 = Index Array(array=string[] ["1", "2", "3", "4", "5", "6", "7", "None"], index=w178) -> (element=w181:string)
        n31 = Index Array(array=string[] ["A", "B", "C"], index=w179) -> (element=w180:string)
        n32 = call "Rate scan Find Offset.vi"("FtHander IN"=w216, "Sumador"=w203, "Max Recorido Dac"=12, "Valor buscado scalers (5000)"=u16 1 ("Valor buscado scalers"), "Error IN"=w215, "Espera acceso USB"=w209, "T Ventana"=w214) -> ("FtHander OUT"=w207:u32, "Todos los valores"=→"Todos los valores":T3, "VALORES START-STOP"=w201:T2, "Error OUT"=w206:errorcluster)  [unwired: 9 in]
        "VALORES START-STOP" <- w201
        n33 = call "Barra puntos.vi"("#N"=w153) -> ("String"=w152:string)  [unwired: 8 in]
        n34 = Unbundle By Name(w201) -> ("SCALER 1 START"=w200:u16, "SCALER 1 STOP"=w199:u16, "THX START"=w198:u16, "THX STOP"=w197:u16, "VHLTH START"=w163:dbl, "VHLTH STOP"=w165:dbl, "Index 1 start"=w191:i32, "Index 1 Stop"=w190:i32, "SCALER 2 START"=w196:u16, "SCALER 2 STOP"=w195:u16, "THX+3 START"=w194:u16, "THX+3 STOP"=w193:u16, "VLLTH START"=w161:dbl, "VLLTH STOP"=w162:dbl, "Index 2 start"=w189:i32, "Index 2 Stop"=w188:i32)
        n35 = Format Into String(format string="Channel %s Adder %s\n%sTotal Errors: %d%s", w181, w180, w152, w154, w152) -> (resulting string=w183:string)  [unwired: 2 in, 1 out]
        n36 = local write "Indicador"(w183) -> ()
        n37 = global read "Global.Salir Ya.vi" "Cancel"() -> (w158:bool)
        n38 = Subtract(x=w165, y=w163) -> (x-y=w172:dbl)
        n39 = Subtract(x=w162, y=w161) -> (x-y=w171:dbl)
        n40 = Divide(x=w171, y=w164) -> (x/y=w170:dbl)
        n41 = Divide(x=w172, y=w164) -> (x/y=w169:dbl)
        n42 = Add(x=w170, y=w161) -> (x+y=w167:dbl)
        n43 = Add(x=w169, y=w163) -> (x+y=w168:dbl)
        n44 = Less?(x=w168, y=w166) -> (x < y?=w160:bool)
        n45 = Less?(x=w167, y=w166) -> (x < y?=w159:bool)
        n46 = Greater Than 0?(x=w154) -> (x > 0?=w155:bool)
        n47 = And(x=w160, y=w159) -> (x .and. y?=w156:bool)
        n48 = Compound Arithmetic op=OR(w156, w158, w155) -> (w157:bool)
      }
      n49 = Increment(x=w117) -> (x+1=w118:i32)
      n50 = Select(t=w117, s=w115, f=w118) -> (s? t:f=w116:i32)
    }
  }
  "Error OUT" <- w73
  n51 = control-ref of="This VI"() -> (w30:refnum<vi>)
  n52 = property class="VI"(reference=w30, "Front Panel.ShowMenuBar"=w33, "TB.Visible"=w33, "Front Panel.TitleBarVis"=TRUE ("Front Panel Window:Title Bar Visible"), "Front Panel.Title"="TEST ASIC. Digital Offset" ("Front Panel Window:Title")) -> ()  [unwired: 1 in, 2 out]
  n53 = call "WINDOWS.AUTO SIZE.vi"("Error In"=w4, "TAB.AutoAjuste"=w29, "This VI"=w30) -> ()  [unwired: 4 in, 1 out]
  n54 = Subtract(x=w48, y=w21) -> (x-y=w46:dbl[][])
  n55 = Subtract(x=w47, y=w20) -> (x-y=w27:dbl[][])
  n56 = Divide(x=w27, y=w26) -> (x/y=w22:dbl[][])
  n57 = Divide(x=w46, y=w26) -> (x/y=w23:dbl[][])
  n58 = Add(x=w22, y=w20) -> (x+y=w24:dbl[][])
  n59 = Add(x=w23, y=w21) -> (x+y=w25:dbl[][])
  n60 = Array Size(array=w25) -> (size(s)=w45:i32[])
  n61 = for {
    tunnel: w19 -> [w222]
    tunnel: w25 -> [w224] mode=indexing
    tunnel: w24 -> [w223] mode=indexing
    tunnel: [w221] -> w41 mode=indexing
    tunnel: [w220] -> w40 mode=indexing
    n62 = Less?(x=w224, y=w222) -> (x < y?=w221:bool[])
    n63 = Less?(x=w223, y=w222) -> (x < y?=w220:bool[])
  }
  n64 = Index Array(array=w45) -> (element #1=w44:i32, element #2=w43:i32)  [unwired: 2 in]
  n65 = Unbundle By Name(w6) -> ("Result"=w65:T9, "Execucion Test.Vasic Actual"=w71:i32)
  n66 = Initialize Array(TRUE, w44, w43) -> (w42:bool[][])
  n67 = Equal?(x=w41, y=w42) -> (x = y?=w58:bool)
  n68 = Equal?(x=w40, y=w42) -> (x = y?=w57:bool)
  n69 = And(x=w58, y=w57) -> (x .and. y?=w39:bool)
  "digital offset all ok" <- w39
  n70 = Index Array(array=w65, index=w71) -> (element=w63:T1)
  n71 = Bundle By Name(cluster=w63, "Test Offset Digital.SCALER 1 START"=w56, "Test Offset Digital.SCALER 1 STOP"=w55, "Test Offset Digital.THX START"=w54, "Test Offset Digital.THX STOP"=w53, "Test Offset Digital.VHLTH START"=w21, "Test Offset Digital.VHLTH STOP"=w48, "Test Offset Digital.Index 1 Start"=w37, "Test Offset Digital.index 1 Stop"=w36, "Test Offset Digital.SCALER 2 START"=w52, "Test Offset Digital.SCALER 2 STOP"=w51, "Test Offset Digital.THX+3 START"=w50, "Test Offset Digital.THX+3 STOP"=w49, "Test Offset Digital.VLLTH START"=w20, "Test Offset Digital.VLLTH STOP"=w47, "Test Offset Digital.Index 2 Start"=w35, "Test Offset Digital.index 2 Stop"=w34, "Test Offset Digital.Ref"=w38, "Test Offset Digital.Offset Digital OK"=w39, "Test Offset Digital.Dig HLTH OK"=w41, "Test Offset Digital.Dig LLTH 2 OK"=w40, "info temp.T Asic Digital Offset"=w7) -> (w11:T1)
  "Result" <- w11
  n72 = Insert Into Array(array=w65, index=w71, new element=w11) -> (w64:T9)
  n73 = Bundle By Name(cluster=w6, "Result"=w64, "Config HW.FT_Handle"=w72) -> (w10:T4)
  "Config Test OUT" <- w10
  n74 = flat-sequence {
    tunnel: w10 -> [_]
    frame #0 {
      n75 = control-ref of="This VI"() -> (w225:refnum<vi>)
      n76 = invoke class="VI" method="FP.Close"(reference=w225) -> ()  [unwired: 2 in, 3 out]
    }
  }
